vi "RSZVB Set TDIF Source Power Mode.vi"(8 "error in (no error)":errorcluster {"code" format="%.0x"}, 9 "Source Power Mode (0: Single-ended)":i32(ring) items=["Single-ended", "Differential and Common Mode"], 10 "Channel (1)":i32=1, 11 "VISA session":refnum<visa-resource-name>) -> (0 "error out":errorcluster {"code" format="%.0x"}, 3 "dup VISA session":refnum<visa-resource-name>)   [LabVIEW 2011]
doc: "This VI qualifies whether the source power (SOURce<Ch>:POWer<Pt>[:LEVel][:IMMediate][:AMPlitude]) is equal to the power of each single-ended wave or to the balanced waves in true differential mode. \n\nNote(s):\n\n(1) This VI is available only with option R&S ZVA-K6 and ZVT instrument.\n\nRemote-control command(s):\nSOURce<Ch>:TDIF:WAVes SENDed | DCMode"
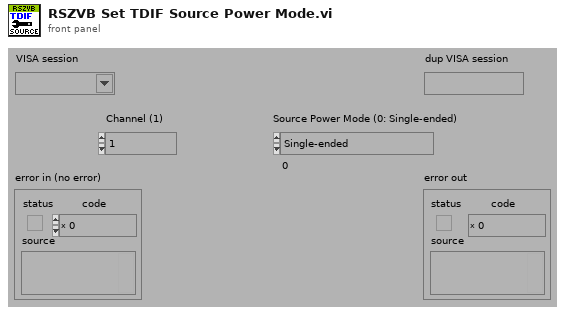
[diagram p1: front panel]
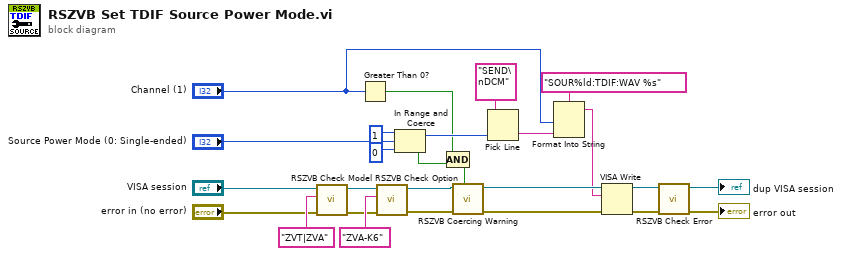
[diagram p0: block diagram]
diagram:
  n1 = call "RSZVB Check Model.vi"("error in (no error)"="error in (no error)", "Model"="ZVT|ZVA" ("Options"), "VISA session"="VISA session") -> ("error out"=w24:errorcluster, "dup VISA session"=w25:refnum<visa-resource-name>)  [unwired: 7 in]
  n2 = Greater Than 0?(x="Channel (1)") -> (x > 0?=w11:bool)
  n3 = call "RSZVB Check Option.vi"("error in (no error)"=w24, "Options"="ZVA-K6", "VISA session"=w25) -> ("error out"=w5:errorcluster, "dup VISA session"=w6:refnum<visa-resource-name>)  [unwired: 7 in]
  n4 = In Range and Coerce(upper limit=1, x="Source Power Mode (0: Single-ended)", lower limit=0) -> (coerced(x)=w19:i32, In Range?=w12:bool)
  n5 = Compound Arithmetic op=AND(w11, w12) -> (w10:bool)
  n6 = call "RSZVB Coercing Warning.vi"("In Range?"=w10, "error in (no error)"=w5, "VISA session"=w6) -> ("error out"=w16:errorcluster, "dup VISA session"=w17:refnum<visa-resource-name>)  [unwired: 7 in]
  n7 = Pick Line(multi-line string="SEND\nDCM", line index=w19) -> (output string=w13:string)  [unwired: 1 in]
  n8 = Format Into String(format string="SOUR%ld:TDIF:WAV %s", "Channel (1)", w13) -> (resulting string=w9:string)  [unwired: 2 in, 1 out]
  n9 = VISA Write(VISA resource name=w17, write buffer=w9, error in (no error)=w16) -> (VISA resource name out=w14:refnum<visa-resource-name>, error out=w15:errorcluster)  [unwired: 1 out]
  n10 = call "RSZVB Check Error.vi"("error in (no error)"=w15, "VISA session"=w14) -> ("error out"=→"error out":errorcluster, "dup VISA session"=→"dup VISA session":refnum<visa-resource-name>)  [unwired: 8 in]
